vi "cm2nm_best_fid_pairing_all_comb.vi"(3 "ReferenceCombinatations":i32[][](array[numeric]), 4 "ReferenceSessionDataSet":T1[](array[typedef]), 5 "CurrentSessionindeces":i32[](array[numeric]), 6 "CurrentSessionDataSet":T1[](array[typedef])) -> (0 "Array of the total error":dbl[](array[numeric]), 1 "IndexRefrenceSession":i32[][](array[numeric]), 2 "IndexCurrentSession":i32[][](array[numeric]))   [LabVIEW 2011]
doc: "Loop through the list of combinations of the reference fiducials. Currently assumes the reference set will have more fiducials than the current set. The combinations are generated outside this vi."
uses:
  cm2nm_coordinate_information_v2.ctl
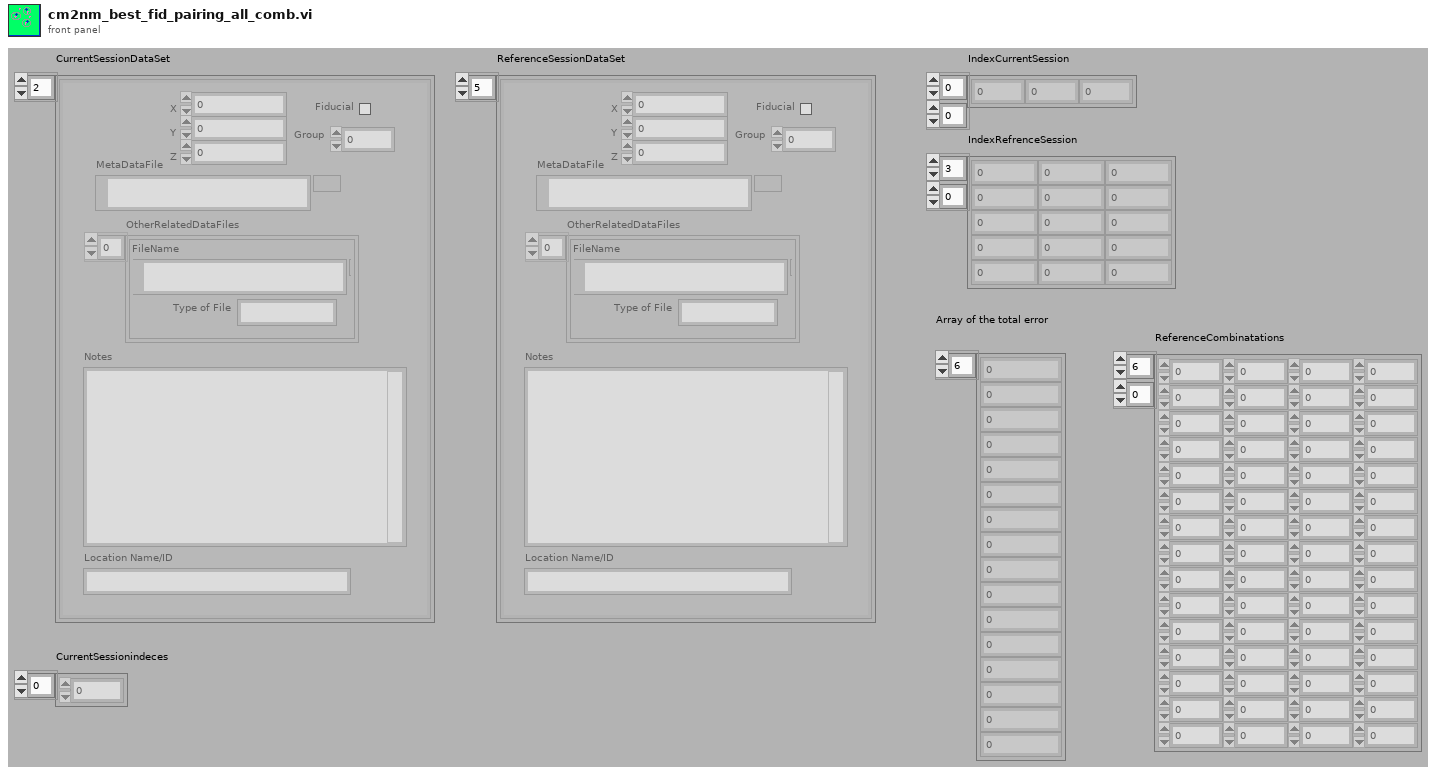
[diagram p1: front panel]
types:
  T1 = typedef "cm2nm_coordinate_information_v2.ctl" = cluster{"MetaDataFile":path, "X":dbl, "Y":dbl, "Z":dbl, "Group":i32, "Rotation":dbl[unit], "Fiducial":bool, "Magnification":dbl, "Working_Distance":dbl, "Notes":string, "Location Name/ID":string, "OtherRelatedDataFiles":cluster{"Type of File":string, "FileName":path}[], "Available":bool}
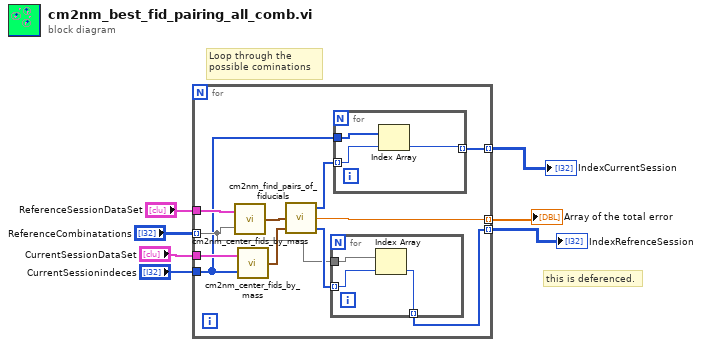
[diagram p0: block diagram]
diagram:
  # "this is deferenced."
  # "Loop through the\npossible cominations"
  n1 = for {
    tunnel: [w12] -> w2 mode=indexing
    tunnel: [w10] -> w7 mode=indexing
    tunnel: "ReferenceSessionDataSet" -> [w18]
    tunnel: "CurrentSessionDataSet" -> [w16]
    tunnel: "CurrentSessionindeces" -> [w8]
    tunnel: "ReferenceCombinatations" -> [w9] mode=indexing
    tunnel: [w14] -> w6 mode=indexing
    n2 = call "cm2nm_center_fids_by_mass.vi"("Array 2"=w9, "CollectionOfPoints"=w18) -> ("Centered and Scaled"=w15:cluster{"X":dbl, "Y":dbl, "Z":dbl}[])
    n3 = call "cm2nm_center_fids_by_mass.vi"("Array 2"=w8, "CollectionOfPoints"=w16) -> ("Centered and Scaled"=w17:cluster{"X":dbl, "Y":dbl, "Z":dbl}[])
    n4 = call "cm2nm_find_pairs_of_fiducials.vi"("CurrentSessionFiducialLocations"=w17, "ReferenceFiducialLocations"=w15) -> ("IndexRefrenceSession"=w11:i32[], "min_distance"=w14:dbl, "IndexCurrentSession"=w13:i32[])  [unwired: 1 in]
    n5 = for {
      tunnel: w11 -> [w20] mode=indexing
      tunnel: w9 -> [w21]
      tunnel: [w19] -> w10 mode=indexing
      n6 = Index Array(array=w21, index=w20) -> (element=w19:i32)
    }
    n7 = for {
      tunnel: w13 -> [w23] mode=indexing
      tunnel: w8 -> [w24]
      tunnel: [w22] -> w12 mode=indexing
      n8 = Index Array(array=w24, index=w23) -> (element=w22:i32)
    }
  }
  "IndexRefrenceSession" <- w7
  "Array of the total error" <- w6
  "IndexCurrentSession" <- w2
